vi "Multiply Polynomials (DBL).vi"(8 "threshold type":T1 items=["Absolute Value", "Relative Value"], 9 "threshold":dbl, 10 "Q(x)":dbl[](array[numeric]), 11 "P(x)":dbl[](array[numeric])) -> (0 "error":i32, 3 "P(x)*Q(x)":dbl[](array[numeric]))   [LabVIEW 2014, in "NI_AALPro.lvlib"]
doc: "Multiplies polynomial <B>P(x)</B> by polynomial <B>Q(x)</B>. The data types you wire to the <B>P(x)</B> and <B>Q(x)</B> inputs determine the polymorphic instance to use."
uses:
  NI_AALPro.lvlib
  Remove Zero Threshold Type.ctl
  1D Convolution (DBL).vi
  Remove Zero Coefficients (DBL).vi
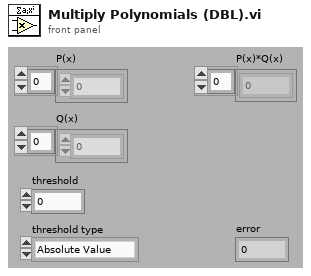
[diagram p1: front panel]
types:
  T1 = typedef "NI_AALPro.lvlib/Remove Zero Threshold Type.ctl" = u16
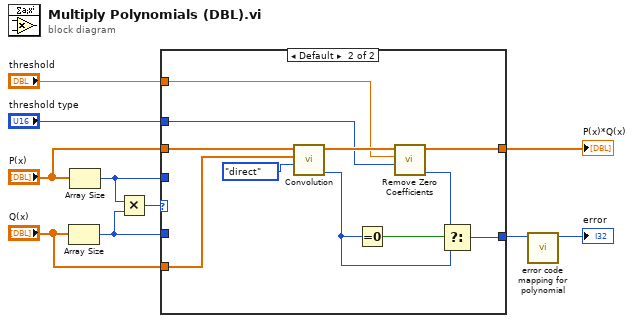
[diagram p0: block diagram]
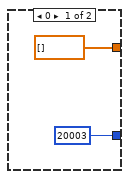
[diagram p2: hidden frame]
diagram:
  n1 = Array Size(array="Q(x)") -> (size(s)=w6:i32)
  n2 = Array Size(array="P(x)") -> (size(s)=w7:i32)
  n3 = Multiply(x=w7, y=w6) -> (x*y=w8:i32)
  n4 = case shown="Default" w8 {
    tunnel: w7 -> [_ _]
    tunnel: w6 -> [_ _]
    tunnel: "P(x)" -> [_ w23]
    tunnel: "Q(x)" -> [_ w22]
    tunnel: [dbl[] [] ("BDL") w16] -> w5
    tunnel: [20003 ("empty array") w18] -> w4
    tunnel: "threshold" -> [_ w14]
    tunnel: "threshold type" -> [_ w13]
    frame 0 {
    }
    frame Default {
      n5 = call-poly "Convolution.vi"("algorithm"=enum32{"direct", "frequency domain"}."direct", "Y"=w22, "X"=w23) -> ("error"=w19:i32, "X * Y"=w17:dbl[])  [unwired: 7 in]
      n6 = Equal To 0?(x=w19) -> (x = 0?=w20:bool)
      n7 = call-poly "Remove Zero Coefficients.vi"("threshold type"=w13, "threshold"=w14, "P(x) In"=w17) -> ("error"=w15:i32, "P(x) Out"=w16:dbl[])  [unwired: 6 in, 1 out]
      n8 = Select(t=w15, s=w20, f=w19) -> (s? t:f=w18:i32)
    }
  }
  "P(x)*Q(x)" <- w5
  n9 = call "error code mapping for polynomial.vi"("error in"=w4) -> ("error out"=→"error":i32)  [unwired: 10 in]
